vi "Initialize Front Panel.vi"(8 "error in":errorcluster, 11 "Peer Review in":refnum<class "Peer Review.lvclass">) -> (0 "error out":errorcluster, 2 "Event Registration Refnum":refnum<event-registration>, 3 "Peer Review out":refnum<class "Peer Review.lvclass">)   [LabVIEW 2020, in "Peer Review.lvclass"]
uses:
  Peer Review.lvclass
  Peer Review.lvclass/Peer Review.ctl
  <vilib>/Utility/miscctls.llb/LVRowAndColumnTypeDef.ctl
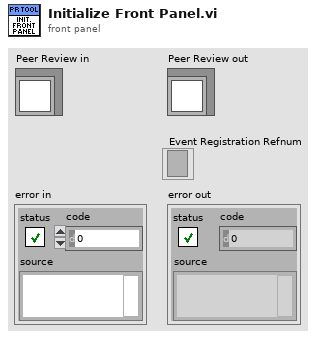
[diagram p1: front panel]
types:
  T1 = typedef "LVRowAndColumnTypeDef.ctl" = cluster{"Row":i32, "Column":i32}
  T2 = enum8{"Enabled", "Disabled", "Disabled and Grayed Out"}
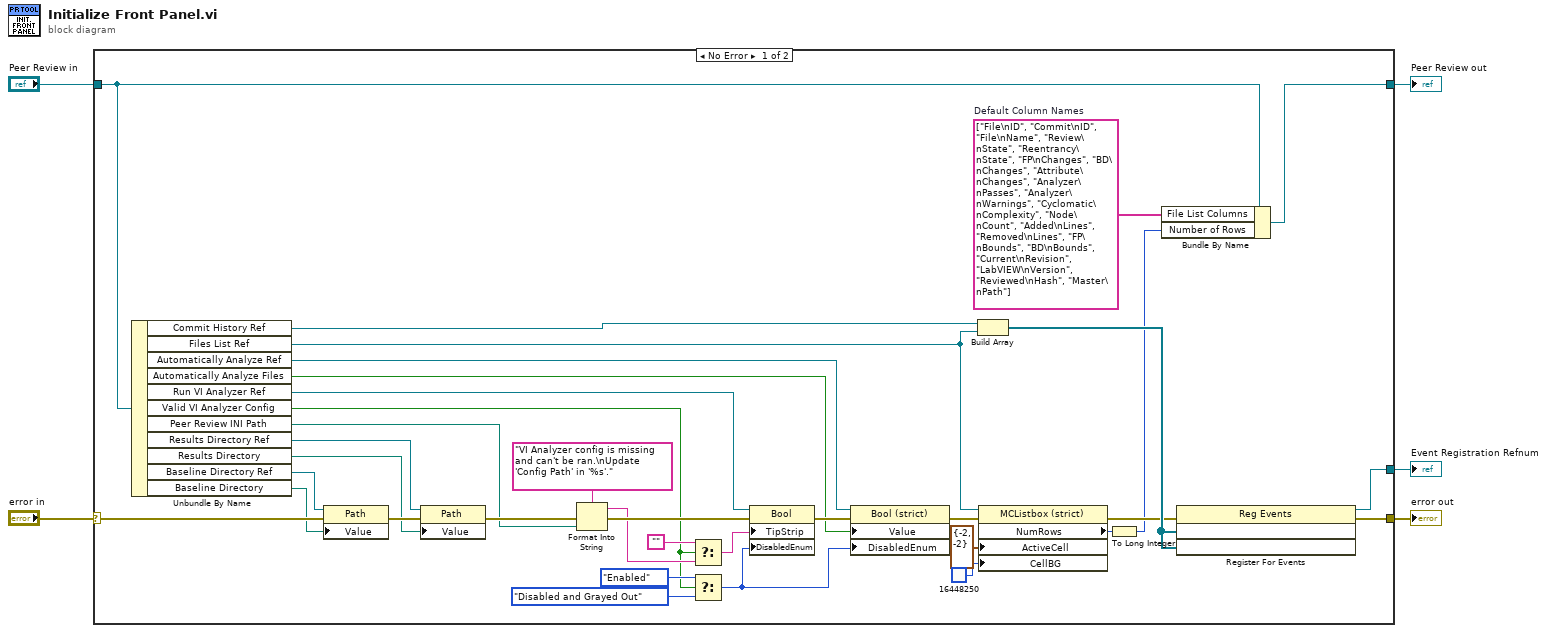
[diagram p0: block diagram]
diagram:
  n1 = case shown="No Error" "error in" {
    selector: "error in" -> [w39 w42]
    tunnel: [w21 w42] -> w4
    tunnel: [w19 w41] -> w2
    tunnel: "Peer Review in" -> [w18 w41]
    tunnel: [w20 _] -> w1
    frame No Error {
      w8 = string[] ["File\nID", "Commit\nID", "File\nName", "Review\nState", "Reentrancy\nState", "FP\nChanges", "BD\nChanges", "Attribute\nChanges", "Analyzer\nPasses", "Analyzer\nWarnings", "Cyclomatic\nComplexity", "Node\nCount", "Added\nLines", "Removed\nLines", "FP\nBounds", "BD\nBounds", "Current\nRevision", "LabVIEW\nVersion", "Reviewed\nHash", "Master\nPath"]  # Default Column Names
      n2 = Unbundle By Name(w18) -> ("Commit History Ref"=w23:refnum<vi>, "Files List Ref"=w10:refnum<vi>, "Automatically Analyze Ref"=w16:refnum<vi>, "Automatically Analyze Files"=w15:bool, "Run VI Analyzer Ref"=w34:refnum<vi>, "Valid VI Analyzer Config"=w24:bool, "Peer Review INI Path"=w22:path, "Results Directory Ref"=w37:refnum<vi>, "Results Directory"=w35:path, "Baseline Directory Ref"=w38:refnum<vi>, "Baseline Directory"=w36:path)
      n3 = property on="Property Node" class="Path"(reference=w38, error in=w39, "Value"=w36) -> (error out=w40:errorcluster)  [unwired: 1 out]
      n4 = property on="Property Node" class="Path"(reference=w37, error in=w40, "Value"=w35) -> (error out=w31:errorcluster)  [unwired: 1 out]
      n5 = Format Into String(format string="VI Analyzer config is missing and can't be ran.\nUpdate 'Config Path' in '%s'." ("f"), error in=w31, w22) -> (resulting string=w26:string, error out=w30:errorcluster)  [unwired: 1 in]
      n6 = Select(t="", s=w24, f=w26) -> (s? t:f=w25:string)
      n7 = Select(t=T2."Enabled" ("Disabled"), s=w24, f=T2."Disabled and Grayed Out" ("Disabled")) -> (s? t:f=w14:T2)
      n8 = property on="Property Node" class="Bool"(reference=w34, error in=w30, "TipStrip"=w25, "DisabledEnum"=w14) -> (error out=w17:errorcluster)  [unwired: 1 out]
      n9 = property on="Property Node" class="Bool (strict)"(reference=w16, error in=w17, "Value"=w15, "DisabledEnum"=w14) -> (error out=w12:errorcluster)  [unwired: 1 out]
      n10 = Build Array(w23, w10) -> (w28:refnum<vi>[])
      n11 = property class="MCListbox (strict)"(reference=w10, error in=w12, "ActiveCell"=T1 {"Row"=-2, "Column"=-2} ("Active Cell:Active Cell"), "CellBG"=u32 16448250) -> (error out=w11:errorcluster, "NumRows"=w13:u32)  [unwired: 1 out]
      n12 = To Long Integer(number=w13) -> (32bit integer=w9:i32)
      n13 = Bundle By Name(cluster=w18, "File List Columns"=w8, "Number of Rows"=w9) -> (w19:refnum<class "Peer Review.lvclass">)
      n14 = register-events(error in=w11, w28, w28) -> (reference out=w20:refnum<event-registration>, error out=w21:errorcluster)  [unwired: 1 in]
    }
    frame Error {
    }
  }
  "error out" <- w4
  "Peer Review out" <- w2
  "Event Registration Refnum" <- w1
